vi "Motors Status.vi"(7 "error in":errorcluster, 8 "VISA in":refnum<visa-resource-name>, 9 "Axis":i32, 10 "Axis Multiplier":i32) -> (0 "error out":errorcluster, 1 "VISA out":refnum<visa-resource-name>, 2 "OS":i32, 3 "Actual Position (mm or deg)":dbl)   [LabVIEW 2018]
panel:
  out "OA buffer":string
  out "OS buffer":string
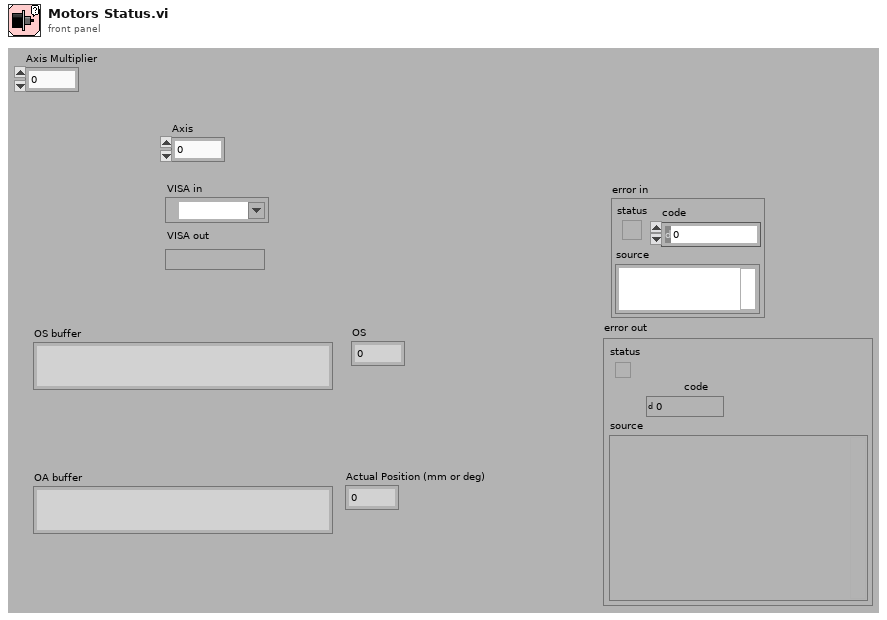
[diagram p1: front panel]
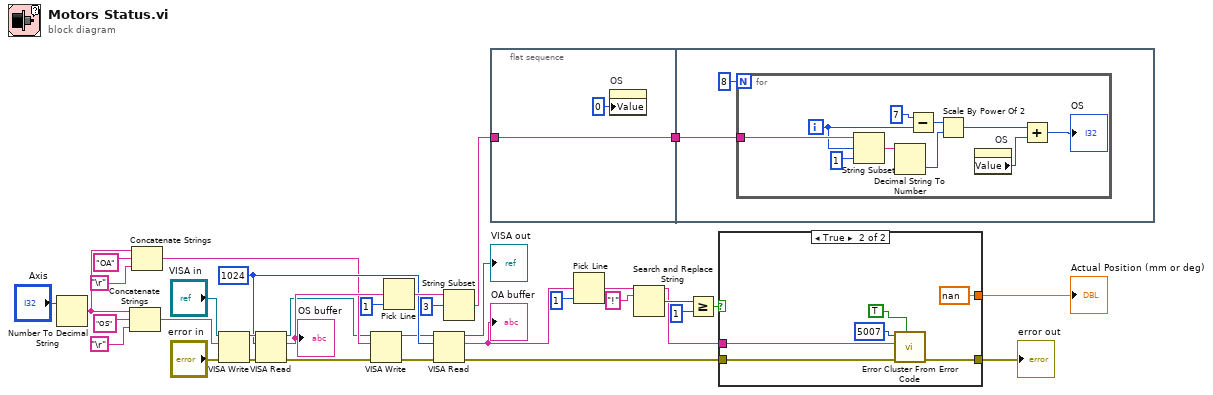
[diagram p0: block diagram]
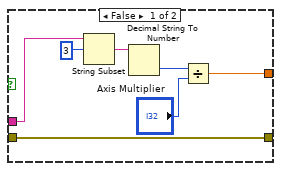
[diagram p2: hidden frame]
diagram:
  w25 = u32 1024 ("byte count")
  n1 = Number To Decimal String(number="Axis") -> (decimal integer string=w18:string)  [unwired: 1 in]
  n2 = Concatenate Strings(w18, "OS" ("Initial command 1"), "\r") -> (w32:string)
  n3 = Concatenate Strings(w18, "OA" ("Initial command 1"), "\r") -> (w17:string)
  n4 = VISA Write(VISA resource name="VISA in", write buffer=w32, error in (no error)="error in") -> (VISA resource name out=w35:refnum<visa-resource-name>, error out=w34:errorcluster)  [unwired: 1 out]
  n5 = VISA Read(VISA resource name=w35, byte count=w25, error in (no error)=w34) -> (VISA resource name out=w10:refnum<visa-resource-name>, read buffer=w30:string, error out=w11:errorcluster)  [unwired: 1 out]
  "OS buffer" <- w30
  n6 = VISA Write(VISA resource name=w10, write buffer=w17, error in (no error)=w11) -> (VISA resource name out=w16:refnum<visa-resource-name>, error out=w15:errorcluster)  [unwired: 1 out]
  n7 = Pick Line(multi-line string=w30, line index=1) -> (output string=w29:string)  [unwired: 1 in]
  n8 = VISA Read(VISA resource name=w16, byte count=w25, error in (no error)=w15) -> (VISA resource name out=→"VISA out":refnum<visa-resource-name>, read buffer=w13:string, error out=w3:errorcluster)  [unwired: 1 out]
  "OA buffer" <- w13
  n9 = String Subset(string=w29, offset (0)=3) -> (substring=w22:string)  [unwired: 1 in]
  n10 = flat-sequence {
    tunnel: w22 -> [w37]
    tunnel: [w37] -> w21
    tunnel: w21 -> [w39]
    frame #0 {
      n11 = property on="OS" class="DigNum (strict)"("Value"=0 ("OS")) -> ()  [unwired: 2 in, 2 out]
    }
    frame #1 {
      n12 = for {
        N: 8 -> [_]
        tunnel: w39 -> [w48]
        i -> [w43]
        n13 = String Subset(string=w48, offset (0)=w43, length (rest)=1 ("length (rest)")) -> (substring=w47:string)
        n14 = Decimal String To Number(string=w47) -> (number=w46:i32)  [unwired: 2 in, 1 out]
        n15 = Subtract(x=7, y=w43) -> (x-y=w45:i32)
        n16 = Scale By Power Of 2(n=w45, x=w46) -> (x*2^n=w42:i32)
        n17 = property on="OS" class="DigNum (strict)"() -> ("Value"=w40:i32)  [unwired: 2 in, 2 out]
        n18 = Add(x=w42, y=w40) -> (x+y=→"OS":i32)
      }
    }
  }
  n19 = Pick Line(multi-line string=w13, line index=1) -> (output string=w5:string)  [unwired: 1 in]
  n20 = Search and Replace String(input string=w5, search string="!") -> (result string=w1:string, number of replacements=w8:i32)  [unwired: 6 in, 2 out]
  n21 = Greater Or Equal?(x=w8, y=1) -> (x >= y?=w6:bool)
  n22 = case shown="True" w6 {
    tunnel: w1 -> [w52 w59]
    tunnel: [w51 w60] -> w4
    tunnel: w3 -> [w51 w61]
    tunnel: [w50 nan] -> w2
    frame False {
      n23 = String Subset(string=w52, offset (0)=3) -> (substring=w54:string)  [unwired: 1 in]
      n24 = Decimal String To Number(string=w54) -> (number=w55:i32)  [unwired: 2 in, 1 out]
      n25 = Divide(x=w55, y="Axis Multiplier") -> (x/y=w50:dbl)
    }
    frame True {
      n26 = call <vilib>:"Error Cluster From Error Code.vi"("show call chain? (False)"=TRUE, "error in (no error)"=w61, "error message (\"\")"=w59, "error code (0)"=5007) -> ("error out"=w60:errorcluster)  [unwired: 5 in]
    }
  }
  "error out" <- w4
  "Actual Position (mm or deg)" <- w2
